vi "Size.vi"(7 "VI Ref":refnum<vi>, 8 "Error":errorcluster, 11 "DecFrame_FP":refnum<class "DecFrame_FP.lvclass">) -> (0 "Error Out":errorcluster, 3 "DecFrame_FP Out":refnum<class "DecFrame_FP.lvclass">, 5 "VI Out":refnum<vi>)   [LabVIEW 2023, in "DecFrame_FP.lvclass"]
uses:
  DecFrame_FP.lvclass
  C:/Users/Mark.Balla/Projects/~FRC/GIT/2024SwerveDrive/2024 Ripon Swerve Source/PC Config/Utility/FP/FPClass/FP/FP.lvclass
  DecFrame_FP.lvclass/DecFrame_FP.ctl
  GObject_FPSZ/GObject_FPSZ.lvclass
  FP/FP.lvclass
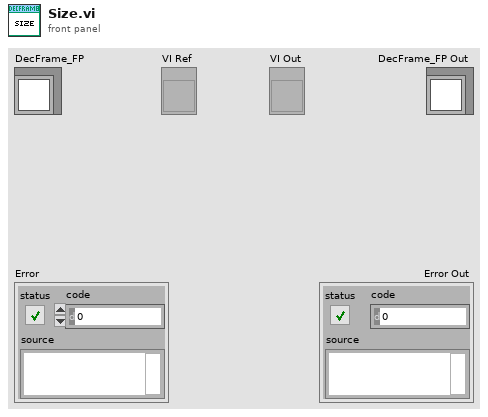
[diagram p1: front panel]
types:
  T1 = typedef "LVRectTypeDef.ctl" = cluster{"Left":i16, "Top":i16, "Right":i16, "Bottom":i16}
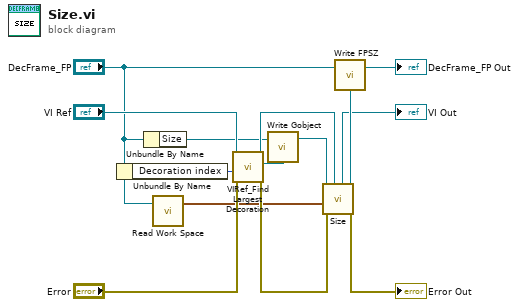
[diagram p0: block diagram]
diagram:
  n1 = Unbundle By Name("DecFrame_FP") -> ("Decoration index"=w7:i32)
  n2 = Unbundle By Name("DecFrame_FP") -> ("Size"=w6:refnum<class "GObject_FPSZ.lvclass">)
  n3 = call "Read Work Space.vi"("FP"="DecFrame_FP") -> ("WkSpace Out"=w1:T1)  [unwired: 2 in]
  n4 = call "VIRef_Find Largest Decoration.vi"("Error"="Error", "Decoration index"=w7, "VI's Ref"="VI Ref") -> ("Error Out"=w5:errorcluster, "Decor Refnum Out"=w13:refnum<vi>, "Calling VI's Ref Out"=w14:refnum<vi>)  [unwired: 2 in, 4 out]
  n5 = call "Write Gobject.vi"("GObject_FPSZ"=w6, "GObj"=w13) -> ("GObject_FPSZ Out"=w12:refnum<class "GObject_FPSZ.lvclass">)  [unwired: 3 in]
  n6 = call-dynamic "Size.vi"("VI"=w14, "Error"=w5, "WkSpace"=w1, "GObject_FPSZ"=w12) -> ("Error Out"=→"Error Out":errorcluster, "GObject_FPSZ Out"=w11:refnum<class "GObject_FPSZ.lvclass">, "VI Out"=→"VI Out":refnum<vi>)  [unwired: 5 in]
  n7 = call "Write FPSZ.vi"("FP"="DecFrame_FP", "FPSZ"=w11) -> ("FP Out"=→"DecFrame_FP Out":refnum<class "DecFrame_FP.lvclass">)  [unwired: 3 in]
